vi "MGI Filter Table Rows.vi"(7 "Illegal Character (\"|\")":string="|", 10 "Column Filters":string[](array[string]), 11 "Table":string[][](array[string])) -> (2 "[Row]":i32[](array[numeric]), 3 "Filtered Table":string[][](array[string]))   [LabVIEW 2020]
doc: "Filters the input table using the specified Column Filters. The implementation depends on the use of an Illegal Character that does not appear in Table or in Column Filters and is not a special character in match pattern (+,*,^,etc).\nThe row index of each match is also output.\n\nColumn Filter values may be:\n<arbitraryText>=Match arbitrary text\n=Match empty Strings\n*=Match anything\n.=Match non-empty strings\n**^<text>=Ends with <text>\n*^*<text>=Contains <text>\n^**<text>=Begins with <text>\n\nAuthored by Shawn Walpole\nsupport@mooregoodideas.com\nwww.mooregoodideas.com\n\nCopyright (c) 2010, Moore Good Ideas, Inc.\n\nAll rights reserved.\n\nRedistribution and use in source and binary forms, with or without modification, are permitted provided that the following conditions are met:\n\n * Redistributions of source code must retain the above copyright notice, this list of conditions and the following disclaimer.\n * Redistributions in binary form must reproduce the above copyright notice, this list of conditions and the following disclaimer in the documentation and/or other materials provided with the distribution.\n * Neither the name of Moore Good Ideas, Inc. nor the names of its contributors may be used to endorse or promote products derived from this software without specific prior written permission.\n\nTHIS SOFTWARE IS PROVIDED BY THE COPYRIGHT HOLDERS AND CONTRIBUTORS \"AS IS\" AND ANY EXPRESS OR IMPLIED WARRANTIES, INCLUDING, BUT NOT LIMITED TO, THE IMPLIED WARRANTIES OF MERCHANTABILITY AND FITNESS FOR A PARTICULAR PURPOSE ARE DISCLAIMED. IN NO EVENT SHALL THE COPYRIGHT OWNER OR CONTRIBUTORS BE LIABLE FOR ANY DIRECT, INDIRECT, INCIDENTAL, SPECIAL, EXEMPLARY, OR CONSEQUENTIAL DAMAGES (INCLUDING, BUT NOT LIMITED TO, PROCUREMENT OF SUBSTITUTE GOODS OR SERVICES; LOSS OF USE, DATA, OR PROFITS; OR BUSINESS INTERRUPTION) HOWEVER CAUSED AND ON ANY THEORY OF LIABILITY, WHETHER IN CONTRACT, STRICT LIABILITY, OR TORT (INCLUDING NEGLIGENCE OR OTHERWISE) ARISING IN ANY WAY OUT OF THE USE OF THIS SOFTWARE, EVEN IF ADVISED OF THE POSSIBILITY OF SUCH DAMAGE."
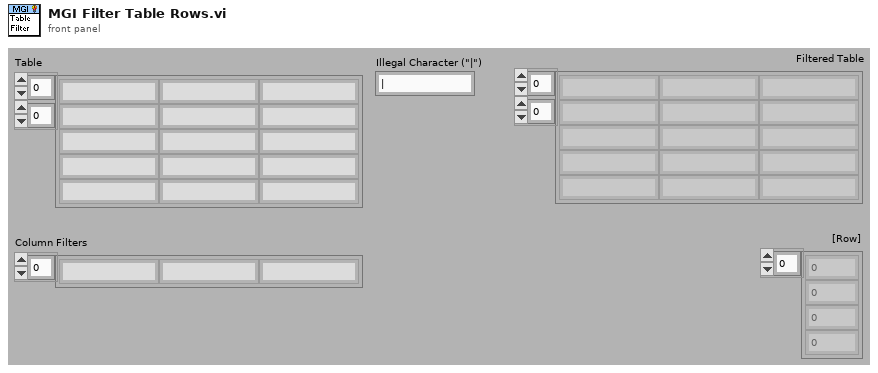
[diagram p1: front panel]
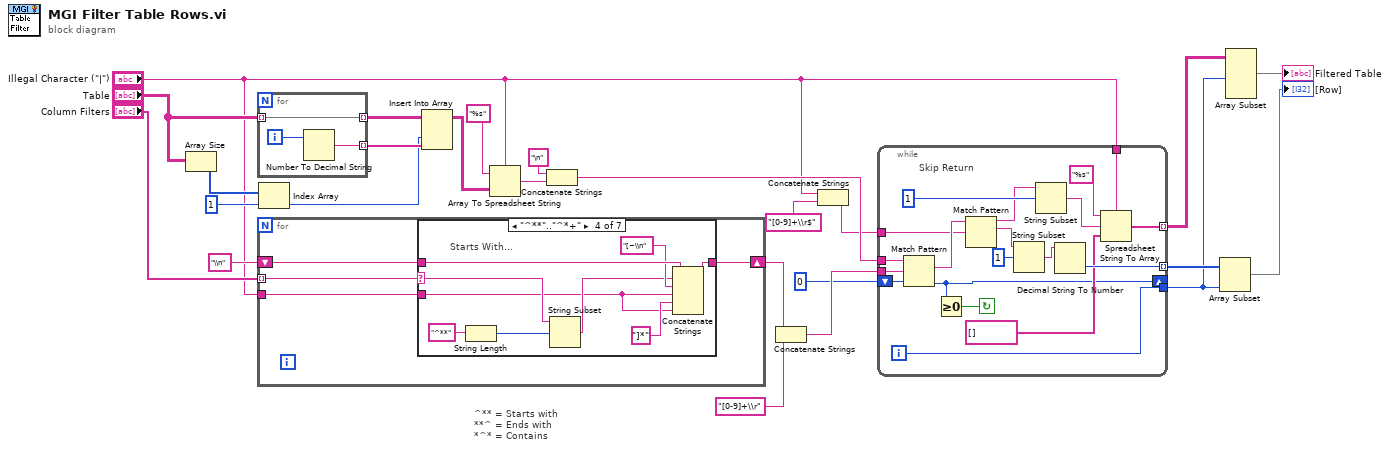
[diagram p0: block diagram]
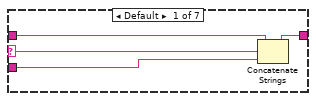
[diagram p2: hidden frame]
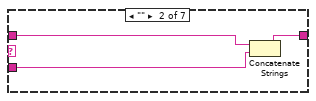
[diagram p3: hidden frame]
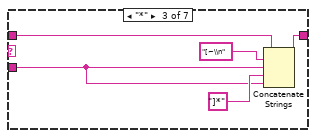
[diagram p4: hidden frame]
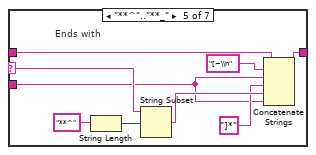
[diagram p5: hidden frame]
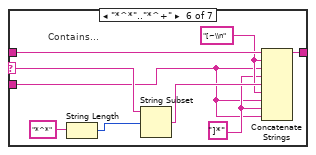
[diagram p6: hidden frame]
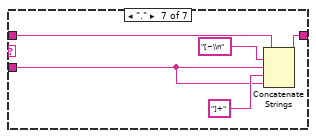
[diagram p7: hidden frame]
diagram:
  # "^** = Starts with\n**^ = Ends with\n*^* = Contains"
  n1 = Array Size(array="Table") -> (size(s)=w7:i32[])
  n2 = for {
    tunnel: "Table" -> [w26] mode=indexing
    tunnel: [w27] -> w16 mode=indexing
    tunnel: [w26] -> w17 mode=indexing
    i -> [w28]
    n3 = Number To Decimal String(number=w28) -> (decimal integer string=w27:string)  [unwired: 1 out]
  }
  n4 = for {
    tunnel: "Column Filters" -> [w30] mode=indexing
    shift-right: [w31] -> w22
    shift-left: "\\n" ("regular expression") -> [w32]
    tunnel: "Illegal Character (\"|\")" -> [w29]
    n5 = case shown="\"^**\"..\"^*+\"" w30 {
      selector: w30 -> [w34 _ _ w50 w60 w69 _]
      tunnel: w32 -> [w36 w39 w44 w53 w62 w71 w76]
      tunnel: [w35 w38 w42 w51 w61 w70 w74] -> w31
      tunnel: w29 -> [w33 w37 w40 w46 w54 w64 w72]
      frame Default {
        n6 = Concatenate Strings(w36, w34, w33) -> (w35:string)
      }
      frame "" {
        n7 = Concatenate Strings(w39, w37) -> (w38:string)
      }
      frame "*" {
        n8 = Concatenate Strings(w44, "[~\\n" ("string"), w40, "]*" ("string"), w40) -> (w42:string)
      }
      frame "^**".."^*+" {
        # "Starts With..."
        n9 = String Length(string="^**") -> (length=w45:i32)
        n10 = String Subset(string=w50, offset (0)=w45) -> (substring=w48:string)  [unwired: 1 out]
        n11 = Concatenate Strings(w53, w48, "[~\\n" ("string"), w46, "]*" ("string"), w46) -> (w51:string)
      }
      frame "**^".."**_" {
        # "Ends with"
        n12 = String Length(string="**^") -> (length=w58:i32)
        n13 = String Subset(string=w60, offset (0)=w58) -> (substring=w56:string)  [unwired: 1 out]
        n14 = Concatenate Strings(w62, "[~\\n" ("string"), w54, "]*" ("string"), w56, w54) -> (w61:string)
      }
      frame "*^*".."*^+" {
        w65 = "]*" ("string")
        w66 = "[~\\n" ("string")
        # "Contains..."
        n15 = String Length(string="*^*") -> (length=w63:i32)
        n16 = String Subset(string=w69, offset (0)=w63) -> (substring=w67:string)  [unwired: 1 out]
        n17 = Concatenate Strings(w71, w66, w64, w65, w67, w66, w64, w65, w64) -> (w70:string)
      }
      frame "." {
        n18 = Concatenate Strings(w76, "[~\\n" ("string"), w72, "]+" ("string"), w72) -> (w74:string)
      }
    }
  }
  n19 = Index Array(array=w7, index=1) -> (element=w5:i32)
  n20 = Insert Into Array(array=w17, index (col)=w5, new element=w16) -> (w15:string[][])  [unwired: 1 in]
  n21 = Array To Spreadsheet String(delimiter (Tab)="Illegal Character (\"|\")", array=w15, 3:"%s" ("format string")) -> (spreadsheet string=w19:string)
  n22 = Concatenate Strings("\n" ("regular expression"), w19) -> (w18:string)
  n23 = Concatenate Strings(w22, "[0-9]+\\r" ("regular expression")) -> (w24:string)
  n24 = Concatenate Strings("Illegal Character (\"|\")", "[0-9]+\\r$" ("regular expression")) -> (w1:string)
  n25 = while {
    shift-right: [w81] -> _
    shift-left: 0 -> [w95]
    tunnel: w24 -> [w93]
    tunnel: w18 -> [w92]
    tunnel: [w88] -> w13 mode=indexing
    tunnel: "Illegal Character (\"|\")" -> [w86]
    tunnel: [w83] -> w11 mode=indexing
    tunnel: [w82] -> w9
    tunnel: w1 -> [w80]
    i -> [w82]
    stop <- w94 continue-if-true
    # "Skip Return"
    n26 = Match Pattern(string=w92, regular expression=w93, offset (0)=w95) -> (match substring=w90:string, offset past match=w81:i32)  [unwired: 2 out]
    n27 = Greater Or Equal To 0?(x=w81) -> (x >= 0?=w94:bool)
    n28 = Match Pattern(string=w90, regular expression=w80) -> (before substring=w89:string, match substring=w79:string)  [unwired: 3 out]
    n29 = String Subset(string=w79, offset (0)=1) -> (substring=w77:string)  [unwired: 1 in]
    n30 = String Subset(string=w89, offset (0)=1) -> (substring=w87:string)  [unwired: 1 in]
    n31 = Decimal String To Number(string=w77) -> (number=w88:i32)  [unwired: 3 out]
    n32 = Spreadsheet String To Array(delimiter (Tab)=w86, format string="%s", spreadsheet string=w87, array type (2D Dbl)=string[] []) -> (array=w83:string[])
  }
  n33 = Array Subset(array=w13, length=w9) -> (→"[Row]":i32[])  [unwired: 1 in]
  n34 = Array Subset(array=w11, length (row)=w9) -> (→"Filtered Table":string[][])  [unwired: 3 in]
